vi "Intent.vi"(8 "error in (no error)":errorcluster, 10 "Intent":T1, 11 "Motions in":refnum<class "Motions.lvclass">) -> (0 "error out":errorcluster, 2 "Actions":T2(array[cluster]), 3 "Motions out":refnum<class "Motions.lvclass">)   [LabVIEW 2016, in "Hardware.lvlib" / "Motions.lvlib" / "Motions.lvclass"]
uses:
  <userlib>/Common Components/Hardware/Abstract System/Motions/Motions/Motions.lvclass
  <userlib>/Common Components/Hardware/Abstract System/Motions/Motions/Motions.lvclass/Motions.ctl
  <userlib>/Common Components/Hardware/Abstract System/Motions/Motions/Intent_Mode_data_UFO.ctl
  <userlib>/Common Components/Hardware/Abstract System/Motions/Motions/Data_Move.ctl
  <userlib>/Common Components/Hardware/Abstract System/Motions/Motions/Data_ENA.ctl
  <vilib>/addons/_JKI.lib/Serialization/JSON/JKI JSON Serialization.lvlib
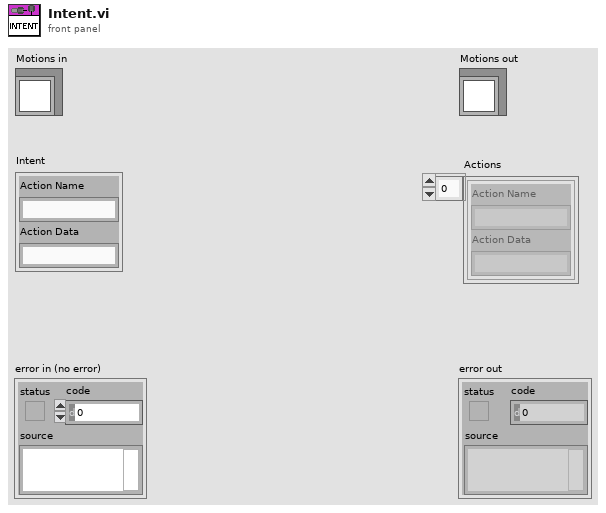
[diagram p1: front panel]
types:
  T1 = cluster{"Action Name":string, "Action Data":string}
  T2 = cluster{"Action Name":string, "Action Data":string}[]
  T3 = typedef "Hardware.lvlib/Motions.lvlib/Motions.lvclass/Intent_Mode.ctl" = enum16{"Default", "XYZ", "UFO"}
  T4 = typedef "Hardware.lvlib/Motions.lvlib/Motions.lvclass/Data_ENA.ctl" = cluster{"Index":i32, "Enable/Disable":bool}
  T5 = typedef "Hardware.lvlib/Motions.lvlib/Motions.lvclass/Intent_Mode_data_UFO.ctl" = cluster{"ROT":u8, "LIN":u8}
  T6 = typedef "Hardware.lvlib/Motions.lvlib/Motions.lvclass/Data_Move.ctl" = cluster{"Index":i32, "Destination":dbl}
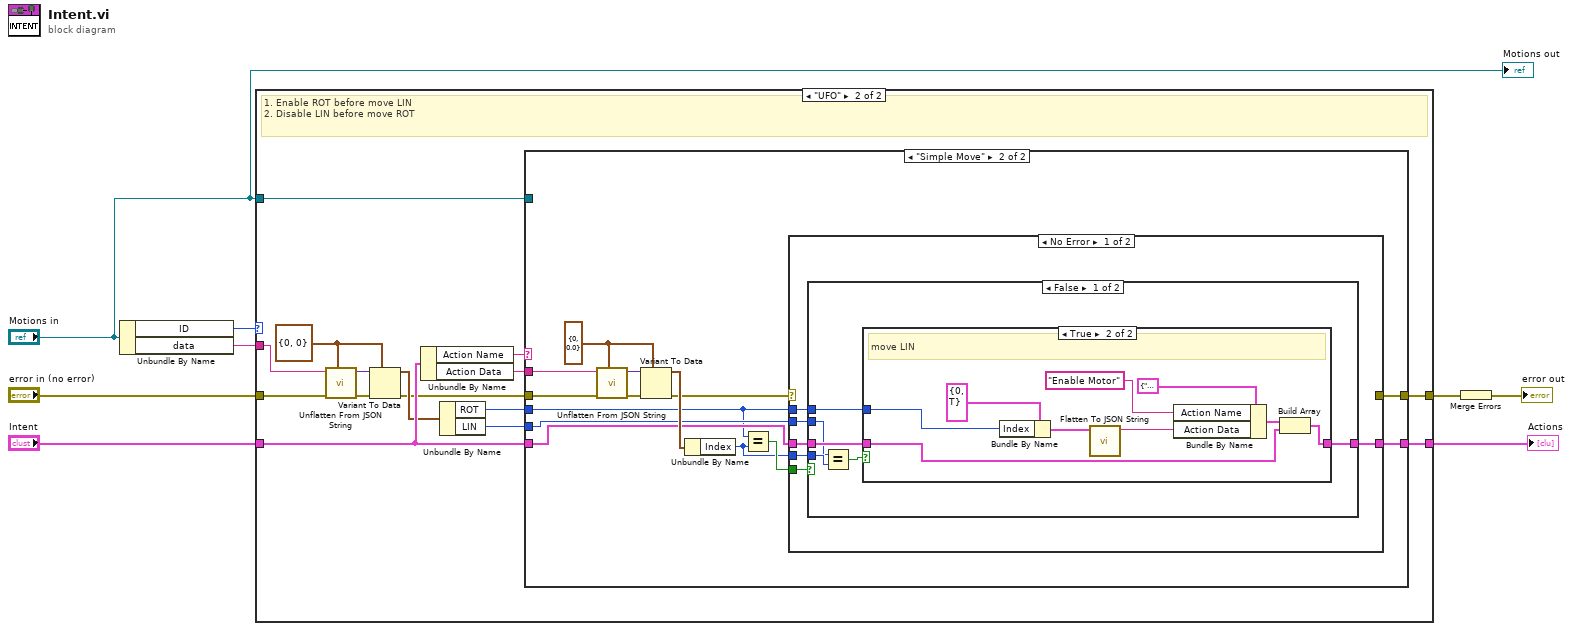
[diagram p0: block diagram]
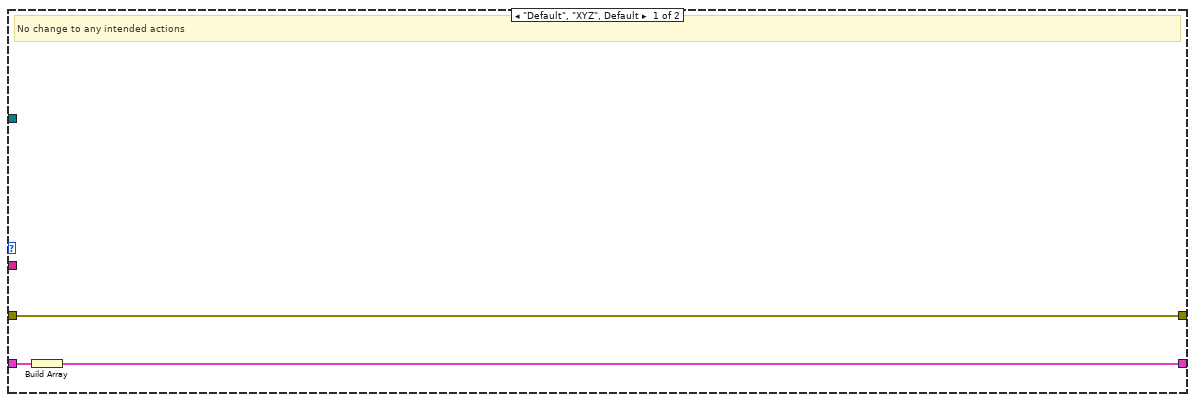
[diagram p2: hidden frame]
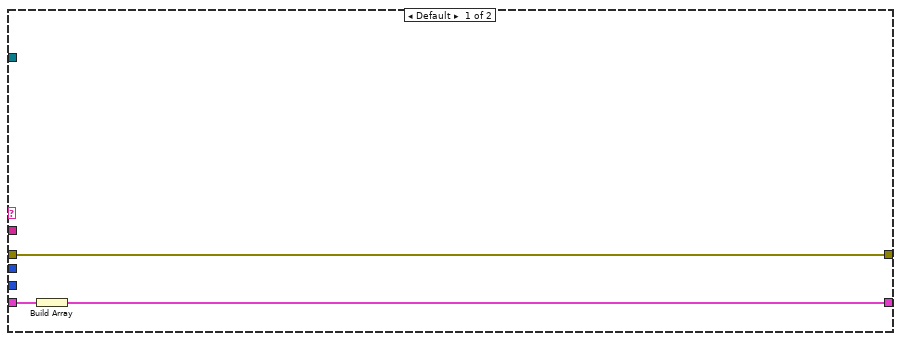
[diagram p3: hidden frame]
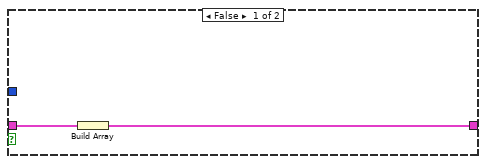
[diagram p4: hidden frame]
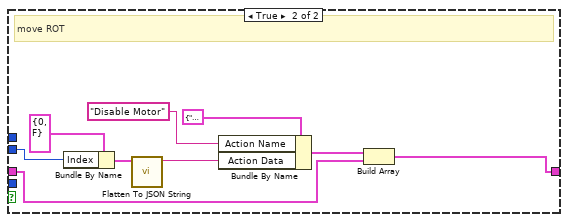
[diagram p5: hidden frame]
diagram:
  n1 = Unbundle By Name("Motions in") -> ("ID"=w2:T3, "data"=w1:string)
  n2 = case shown="\"UFO\"" w2 {
    tunnel: "error in (no error)" -> [w9 w16]
    tunnel: [w9 w26] -> w7
    tunnel: [w10 w23] -> w5
    tunnel: "Intent" -> [w11 w22]
    tunnel: "Motions in" -> [_ w21]
    tunnel: w1 -> [_ w20]
    frame "Default", "XYZ", Default {
      # "No change to any intended actions"
      n3 = Build Array(w11) -> (w10:T2)
    }
    frame "UFO" {
      w18 = T5 {"ROT"=0, "LIN"=0} ("UFO Intent Mode data")
      # "1. Enable ROT before move LIN\n2. Disable LIN before move ROT"
      n4 = call <vilib>:"Unflatten From JSON String.vi"("Type and Defaults"=w18, "error in (no error)"=w16, "JSON String"=w20) -> ("error out"=w15:errorcluster, "Variant"=w19:variant)  [unwired: 7 in]
      n5 = Variant To Data(error in=w15, type=w18, Variant=w19) -> (data=w17:T5, error out=w14:errorcluster)
      n6 = Unbundle By Name(w22) -> ("Action Name"=w25:string, "Action Data"=w24:string)
      n7 = Unbundle By Name(w17) -> ("ROT"=w13:u8, "LIN"=w12:u8)
      n8 = case shown="\"Simple Move\"" w25 {
        tunnel: [w29 w31] -> w26
        tunnel: w24 -> [_ w39]
        tunnel: w14 -> [w29 w41]
        tunnel: [w27 w36] -> w23
        tunnel: w22 -> [w28 w37]
        tunnel: w21 -> [_ _]
        tunnel: w13 -> [_ w30]
        tunnel: w12 -> [_ w33]
        frame Default {
          n9 = Build Array(w28) -> (w27:T2)
        }
        frame "Simple Move" {
          w40 = T6 {"Index"=0, "Destination"=0.0} ("Set Motion Status Data cluster")
          n10 = call <vilib>:"Unflatten From JSON String.vi"("Type and Defaults"=w40, "error in (no error)"=w41, "JSON String"=w39) -> ("error out"=w42:errorcluster, "Variant"=w43:variant)  [unwired: 7 in]
          n11 = Variant To Data(error in=w42, type=w40, Variant=w43) -> (data=w38:T6, error out=w32:errorcluster)
          n12 = Unbundle By Name(w38) -> ("Index"=w34:i32)
          n13 = Equal?(x=w30, y=w34) -> (x = y?=w35:bool)
          n14 = case shown="No Error" w32 {
            selector: w32 -> [_ w76]
            tunnel: w37 -> [w49 _]
            tunnel: [w48 _] -> w36
            tunnel: w35 -> [w47 _]
            tunnel: w34 -> [w46 _]
            tunnel: w33 -> [w45 _]
            tunnel: [_ w76] -> w31
            tunnel: w30 -> [w44 _]
            frame No Error {
              n15 = case shown="False" w47 {
                tunnel: w49 -> [w55 w75]
                tunnel: [w54 w74] -> w48
                tunnel: w46 -> [w53 _]
                tunnel: w45 -> [w52 w69]
                tunnel: w44 -> [w50 _]
                frame False {
                  n16 = Equal?(x=w52, y=w53) -> (x = y?=w51:bool)
                  n17 = case shown="True" w51 {
                    tunnel: w55 -> [w57 w66]
                    tunnel: [w56 w65] -> w54
                    tunnel: w50 -> [_ w60]
                    frame False {
                      n18 = Build Array(w57) -> (w56:T2)
                    }
                    frame True {
                      # "move LIN"
                      n19 = Bundle By Name(cluster=T4 {"Index"=0, "Enable/Disable"=TRUE} ("Set Motion Status Data cluster"), "Index"=w60) -> (w63:T4)
                      n20 = call <vilib>:"Flatten To JSON String.vi"("Variant"=w63) -> ("JSON String"=w62:string)  [unwired: 9 in, 1 out]
                      n21 = Bundle By Name(cluster=T1 {"Action Name"="", "Action Data"=""} ("Intent"), "Action Name"="Enable Motor", "Action Data"=w62) -> (w58:T1)
                      n22 = Build Array(w58, w66) -> (w65:T2)
                    }
                  }
                }
                frame True {
                  # "move ROT"
                  n23 = Bundle By Name(cluster=T4 {"Index"=0, "Enable/Disable"=FALSE} ("Set Motion Status Data cluster"), "Index"=w69) -> (w68:T4)
                  n24 = call <vilib>:"Flatten To JSON String.vi"("Variant"=w68) -> ("JSON String"=w67:string)  [unwired: 9 in, 1 out]
                  n25 = Bundle By Name(cluster=T1 {"Action Name"="", "Action Data"=""} ("Intent"), "Action Name"="Disable Motor", "Action Data"=w67) -> (w72:T1)
                  n26 = Build Array(w72, w75) -> (w74:T2)
                }
              }
            }
            frame Error {
              # "no action on error"
            }
          }
        }
      }
    }
  }
  "Actions" <- w5
  n27 = Merge Errors(w7) -> (→"error out":errorcluster)
  "Motions out" <- "Motions in"
